vi "LINX Analog Read Benchmark.vi"(0 "Stop Button":bool, 11 "AI Channels":u8[](array[numeric])=[0, 0, 0, 0, 0, 0, 0, 0, 0, 0, 0, 0]) -> (2 "Voltages":dbl[](array[numeric])=[1.2665039062499999, 1.26328125, 1.26328125, 1.2665039062499999, 1.2665039062499999, 1.26328125, 1.2665039062499999, 1.26328125, 1.2665039062499999, 1.2665039062499999, 1.2665039062499999, 1.26328125], 3 "Loop Time (ms)":dbl=1.5 format="%#_2g", 6 "Loop Rate":dbl(graph)=1.5)   [LabVIEW 2013]
uses:
  <vilib>/LabVIEW Hacker/LINX/Private/Device/Type Defs/TCP Config.ctl
  <vilib>/LabVIEW Hacker/LINX/Private/Type Defs/Interface.ctl
  <vilib>/LabVIEW Hacker/LINX/Public/Peripherals/Analog/Analog Read N Chans.vi
  <vilib>/ptbypt/NI_PtbyPt.lvlib
  <vilib>/LabVIEW Hacker/LINX/LVH-LINX.lvlib
  <vilib>/LabVIEW Hacker/LINX/Private/Device/Device.lvlib
panel:
  out "Error Out":errorcluster
  in  "COM Port":refnum<visa-resource-name>="COM7"
  in  "Delay":u32
  in  "Interface":T1=enum."TCP"
  in  "TCP Configuration":T2={"IP Address"="10.2.106.213", "Port"=6921}
  out "Voltages":dbl[](graph)=[1.2665039062499999, 1.26328125, 1.26328125, 1.2665039062499999, 1.2665039062499999, 1.26328125, 1.2665039062499999, 1.26328125, 1.2665039062499999, 1.2665039062499999, 1.2665039062499999, 1.26328125]
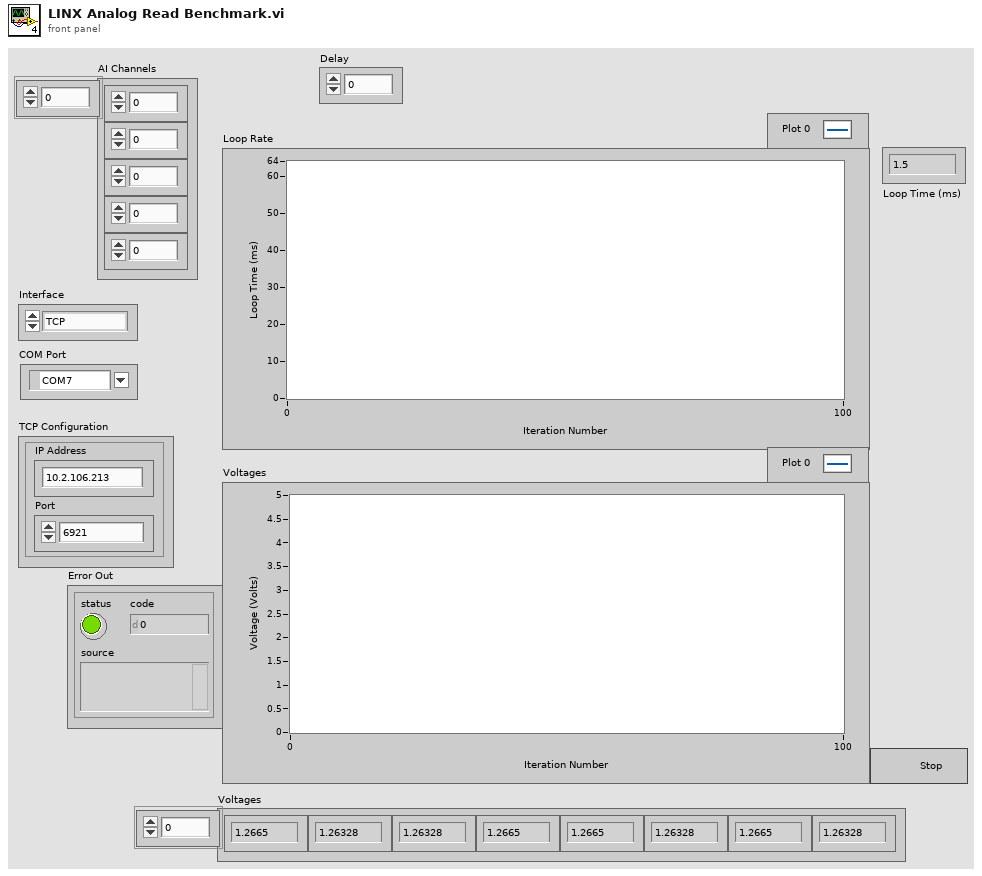
[diagram p1: front panel]
types:
  T1 = typedef "LVH-LINX.lvlib/Interface.ctl" = enum16{"Serial", "TCP"}
  T2 = typedef "LVH-LINX.lvlib/Device.lvlib/TCP Config.ctl" = cluster{"IP Address":string, "Port":u16}
  T3 = typedef "LVH-LINX.lvlib/LINX Ref.ctl" = cluster{"Platform":T4, "Interface":T1, "LINX Device Config":T5}
  T4 = typedef "LVH-LINX.lvlib/Platform.ctl" = enum16{"LINX", "myRIO"}
  T5 = typedef "LVH-LINX.lvlib/Device.lvlib/LINX Device Config.ctl" = cluster{"Interface":T1, "COM Port":refnum<visa-resource-name>, "TCP Configuration":T2, "Device Family":T6, "Device ID":u8, "Device Name":string, "TCP Ref":refnum<k5>}
  T6 = typedef "LVH-LINX.lvlib/Device Family.ctl" = enum8{"National Instruments", "Digilent", "Arduino"}
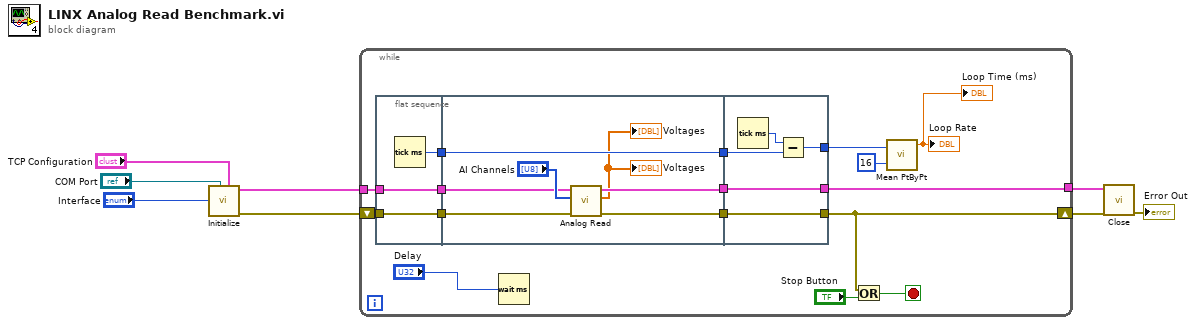
[diagram p0: block diagram]
diagram:
  n1 = call <vilib>:"Initialize.vi"("TCP Configuration"="TCP Configuration", "Serial Port"="COM Port", "Interface"="Interface") -> ("Error Out"=w7:errorcluster, "LINX Ref"=w8:T3)  [unwired: 6 in, 1 out]
  n2 = while {
    tunnel: w8 -> [w24]
    shift-right: [w10] -> w5
    shift-left: w7 -> [w12]
    tunnel: [w15] -> w6
    stop <- w23 stop-if-true
    n3 = flat-sequence {
      tunnel: w24 -> [w27]
      tunnel: [w27] -> w21
      tunnel: [w26] -> w20
      tunnel: w12 -> [w25]
      tunnel: [w25] -> w11
      tunnel: w21 -> [w29]
      tunnel: w20 -> [w34]
      tunnel: [w34] -> w19
      tunnel: [w33] -> w14
      tunnel: [w32] -> w13
      tunnel: w11 -> [w31]
      tunnel: w19 -> [w38]
      tunnel: [w37] -> w18
      tunnel: [w36] -> w15
      tunnel: w14 -> [w36]
      tunnel: w13 -> [w35]
      tunnel: [w35] -> w10
      frame #0 {
        n4 = Tick Count (ms)() -> (millisecond timer value=w26:u32)
      }
      frame #1 {
        n5 = call-poly <vilib>:"Analog Read.vi"("Error In"=w31, "AI Channel(s)"="AI Channels", "LINX Resource"=w29) -> ("Error Out"=w32:errorcluster, "Voltages"=→"Voltages" →"Voltages":dbl[], "LINX Resource"=w33:T3)  [unwired: 5 in, 1 out]
      }
      frame #2 {
        n6 = Tick Count (ms)() -> (millisecond timer value=w39:u32)
        n7 = Subtract(x=w39, y=w38) -> (x-y=w37:u32)
      }
    }
    n8 = Wait (ms)(milliseconds to wait="Delay") -> ()  [unwired: 1 out]
    n9 = Or(x=w10, y="Stop Button") -> (x .or. y?=w23:bool)
    n10 = call <vilib>:"Mean PtByPt.vi"("x"=w18, "sample length"=16) -> ("mean"=→"Loop Rate" →"Loop Time (ms)":dbl)  [unwired: 2 in, 1 out]
  }
  n11 = call <vilib>:"Close.vi"("Error In"=w5, "LINX Resource"=w6) -> ("Error Out"=→"Error Out":errorcluster)  [unwired: 8 in, 1 out]
